vi "Set_Channel_Coeff_server.vi"(0 "Set Array":T1(array[cluster]) {"Set value of D to" format="%.2f"; "Set value of C to" format="%.2f"; "Set value of B to" format="%.2f"; "Set value of A to" format="%.2f"}) -> ()   [LabVIEW 2010]
uses:
  ADAM_Global.vi
  Sub VI's/Channel_Description_Global.vi
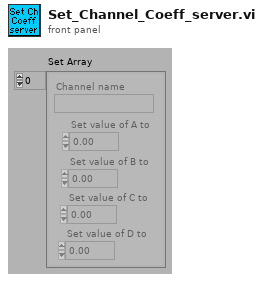
[diagram p1: front panel]
types:
  T1 = cluster{"Channel name":string, "Set value of A to":dbl, "Set value of B to":dbl, "Set value of C to":dbl, "Set value of D to":dbl}[]
  T2 = enum16{"Append to Global", "Read Global then Clear"}
  T3 = typedef "Ch_description_ADAM.ctl" = cluster{"Ch Name":string, "Type":T4, "Function":T5, "Ch State":T6, "Calibration type":T7, "A":dbl, "B":dbl, "C":dbl, "D":dbl, "Comments":string, "Address":T8, "String":string, "Duty":u16}
  T4 = typedef "Module_type_ADAM.ctl" = enum16{"4011", "4012", "4013", "4014", "4016", "4017", "4018", "4021", "4050", "4052", "4053", "4060", "4080", "5000", "5017", "5018", "5024", "5051", "5056", "5060", "6060", "Tracker", "WEST", "GILL", "JEM", "VICI", "Vaisala", "DRUCK", "Run VI Named:", "IR2100", "PPT", "Comparator", "VIRTUAL", "Hold Value", "Read A", "Read Ch", "Coded", "Client Info", "Web Client", "X10", "Test"}
  T5 = typedef "Function_ADAM.ctl" = enum16{"Analogue Input", "Digital Input", "Event counter", "Event rate", "Analogue Output", "Digital Output", "Relay Output"}
  T6 = typedef "Channel_State.ctl" = enum16{"On", "Off", "Always On", "Always Off"}
  T7 = typedef "Calib_type_ADAM.ctl" = enum16{"Raw", "Bx + A", "Cx^2 + Bx + A", "Dx^3 + Cx^2 + Bx + A", "In Band", "Hi-Tec Q", "Hi-Tec M_dot", "Text"}
  T8 = typedef "Address.ctl" = cluster{"Main":i32, "Ch.":i32, "Sub":i32, "Port Name":string}
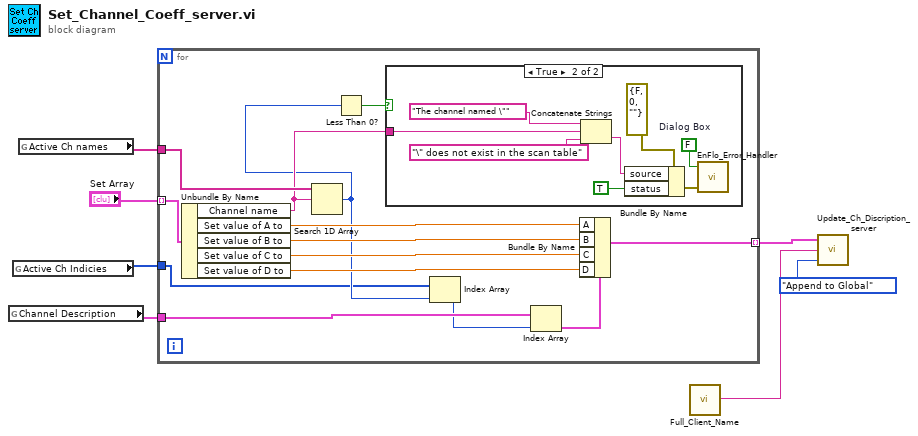
[diagram p0: block diagram]
diagram:
  n1 = global read "Channel_Description_Global.vi" "Channel Description"() -> (w2:T3[])
  n2 = global read "ADAM_Global.vi" "Active Ch Indicies"() -> (w6:i32[])
  n3 = global read "ADAM_Global.vi" "Active Ch names"() -> (w5:string[])
  n4 = for {
    tunnel: w5 -> [w21]
    tunnel: "Set Array" -> [w20] mode=indexing
    tunnel: w2 -> [w12]
    tunnel: w6 -> [w10]
    tunnel: [w8] -> w4 mode=indexing
    n5 = Unbundle By Name(w20) -> ("Channel name"=w14:string, "Set value of A to"=w18:dbl, "Set value of B to"=w17:dbl, "Set value of C to"=w16:dbl, "Set value of D to"=w15:dbl)
    n6 = Search 1D Array(1D array=w21, element=w14) -> (index of element=w11:i32)  [unwired: 1 out]
    n7 = Less Than 0?(x=w11) -> (x < 0?=w13:bool)
    n8 = case shown="True" w13 {
      tunnel: w14 -> [_ w27]
      frame False {
      }
      frame True {
        w22 = FALSE  # Dialog Box
        n9 = Concatenate Strings("The channel named \"", w27, "\" does not exist in the scan table") -> (w24:string)
        n10 = Bundle By Name(cluster=errorcluster {"status"=FALSE, "code"=0, "source"=""} ("error in (no error)"), "source"=w24, "status"=TRUE ("Bundle Element")) -> (w25:errorcluster)
        n11 = call "EnFlo_Error_Handler.vi"("error in (no error)"=w25, "Dialog Box (T)"=w22) -> ()  [unwired: 1 in, 3 out]
      }
    }
    n12 = Index Array(array=w10, index=w11) -> (element=w9:i32)
    n13 = Index Array(array=w12, index=w9) -> (element=w19:T3)
    n14 = Bundle By Name(cluster=w19, "A"=w18, "B"=w17, "C"=w16, "D"=w15) -> (w8:T3)
  }
  n15 = call "Full_Client_Name.vi"() -> ("Client Name"=w1:string)
  n16 = call "Update_Ch_Discription_server.vi"("Mode"=T2."Append to Global", "Client HD name"=w1, "Channels to update In"=w4) -> ()  [unwired: 1 out]
